vi "Create Proto Parser.vi"(8 "error in (no error)":errorcluster) -> (0 "error out":errorcluster, 3 "protoFile ref out":u64)   [LabVIEW 2019, in "gRPC Template Creation Utility.lvlib"]
uses:
  gRPC Template Creation Utility.lvlib
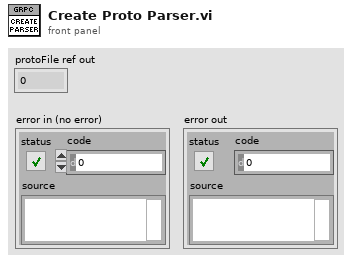
[diagram p1: front panel]
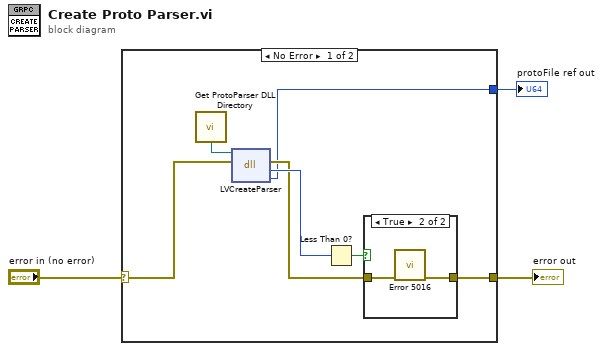
[diagram p0: block diagram]
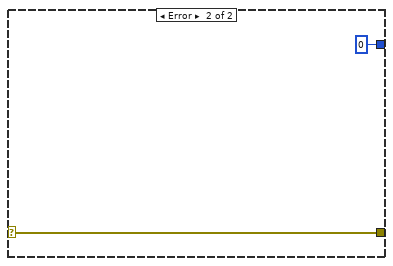
[diagram p3: hidden frame]
diagram:
  n1 = case shown="No Error" "error in (no error)" {
    selector: "error in (no error)" -> [w9 w15]
    tunnel: [w5 w15] -> w3
    tunnel: [w4 u64 0 ("protoRef")] -> w1
    frame No Error {
      n2 = call "Get ProtoParser DLL Directory.vi"() -> ("Proto Parser Directory"=w10:path)
      n3 = dll-call lib="?" fn="LVCreateParser"(path in=w10, error in=w9) -> (error out=w6:errorcluster, "return type"=w8:i32, "protoRef"=w4:u64)  [unwired: 2 in, 1 out]
      n4 = Less Than 0?(x=w8) -> (x < 0?=w7:bool)
      n5 = case shown="True" w7 {
        tunnel: w6 -> [w11 w13]
        tunnel: [w11 w12] -> w5
        frame False {
        }
        frame True {
          n6 = call "Error 5016.vi"("error in (no error)"=w13) -> ("error out"=w12:errorcluster)  [unwired: 10 in]
        }
      }
    }
    frame Error {
    }
  }
  "protoFile ref out" <- w1
  "error out" <- w3
